vi "Acq-module5761.vi"(4 "NumChannels":u16, 5 "DMA number":i32, 6 "Selected Channels":T1[](array[typedef])=[enum."Empty", enum."Empty", enum."Empty", enum."Empty"], 7 "IntermediateFIFO":refnum<k21>="FIFO0", 8 "DebugActivation":bool, 9 "GroupEnableN":bool, 10 "SamplingRateN(DecimationFactor)":u16, 11 "DMATtoHOSTBlockNWords":u16) -> ()   [LabVIEW 2013, in "IRIO.lvlib"]
uses:
  IRIO.lvlib
  ctl/SelectedChannels.ctl
  <vilib>/rvi/DataTransferAndStorage/Container/Common/niFpgaContainerGetUniqueNameForEmu.vi
  <vilib>/rvi/DataTransferAndStorage/Container/Common/niFpgaContainerSetEmuInfo.vi
  <vilib>/rvi/eio/common/nirviEmuReportErrorAndStop.vi
  <vilib>/rvi/DataTransferAndStorage/Container/Common/niFpgaContainerExecOnDevCompGetState.vi
  <vilib>/rvi/DataTransferAndStorage/Register/Emulation/niFpgaRegisterEmulationFpgaImpl.vi
  <instcachedir>/1/niFpgaRegisterEmulationFpgaImpl_DCF4BC0110594B98B44A971D60CEEC4D.lvgen/niFpgaRegisterEmulationFpgaImpl_DCF4BC0110594B98B44A971D60CEEC4D_003.vi
  <instcachedir>/1/niFpgaRegisterEmulationFpgaImpl_DCF4BC0110594B98B44A971D60CEEC4D.lvgen/niFpgaRegisterEmulationFpgaImpl_DCF4BC0110594B98B44A971D60CEEC4D_005.vi
  <vilib>/rvi/eio/common/nirviEmuTemplateMethod_errors.vi
  common/GlobalReg.vi
  <instcachedir>/1/niFpgaRegisterEmulationFpgaImpl_DCF4BC0110594B98B44A971D60CEEC4D.lvgen/niFpgaRegisterEmulationFpgaImpl_DCF4BC0110594B98B44A971D60CEEC4D_004.vi
  <vilib>/rvi/FIFO/Fifo_Resource/nirvififoEmulationWriteFpgaImpl.vi
  <vilib>/rvi/interface/RandomDataEmulation/nirviRandomDataFPGAFIFO.vi
  <vilib>/rvi/interface/RandomDataEmulation/niFpgaRandomDataHandleErrors.vi
  <vilib>/rvi/Emulation/niFpgaSctlEmulationGetInTimedLoop.vi
  <vilib>/rvi/Emulation/niFpgaProcessEmulError.vi
  <vilib>/rvi/LocalResourceManager/LocalResourceManager.xnode
  <vilib>/rvi/DataTransferAndStorage/Container/XNode/niFpgaContainer.xnode
  <vilib>/rvi/DataTransferAndStorage/Register/Emulation/niFpgaRegisterEmulationRefIn.vi
  <vilib>/eio/EIONode/EIONode.xnode
  <vilib>/rvi/FIFO/Fifo_Resource/niFpgaFifoEmulationRefIn.vi
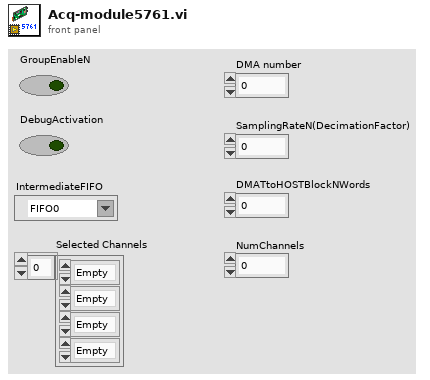
[diagram p1: front panel]
types:
  T1 = typedef "IRIO.lvlib/SelectedChannels.ctl" = enum16{"Empty", "AI0", "AI1", "AI2", "AI3", "SignalGenerator0", "SignalGenerator1", "DDCA_PORT0", "DDCA_PORT1", "DDCA_PORT2", "DDCB_PORT0", "DDCB_PORT1", "DDCB_PORT2"}
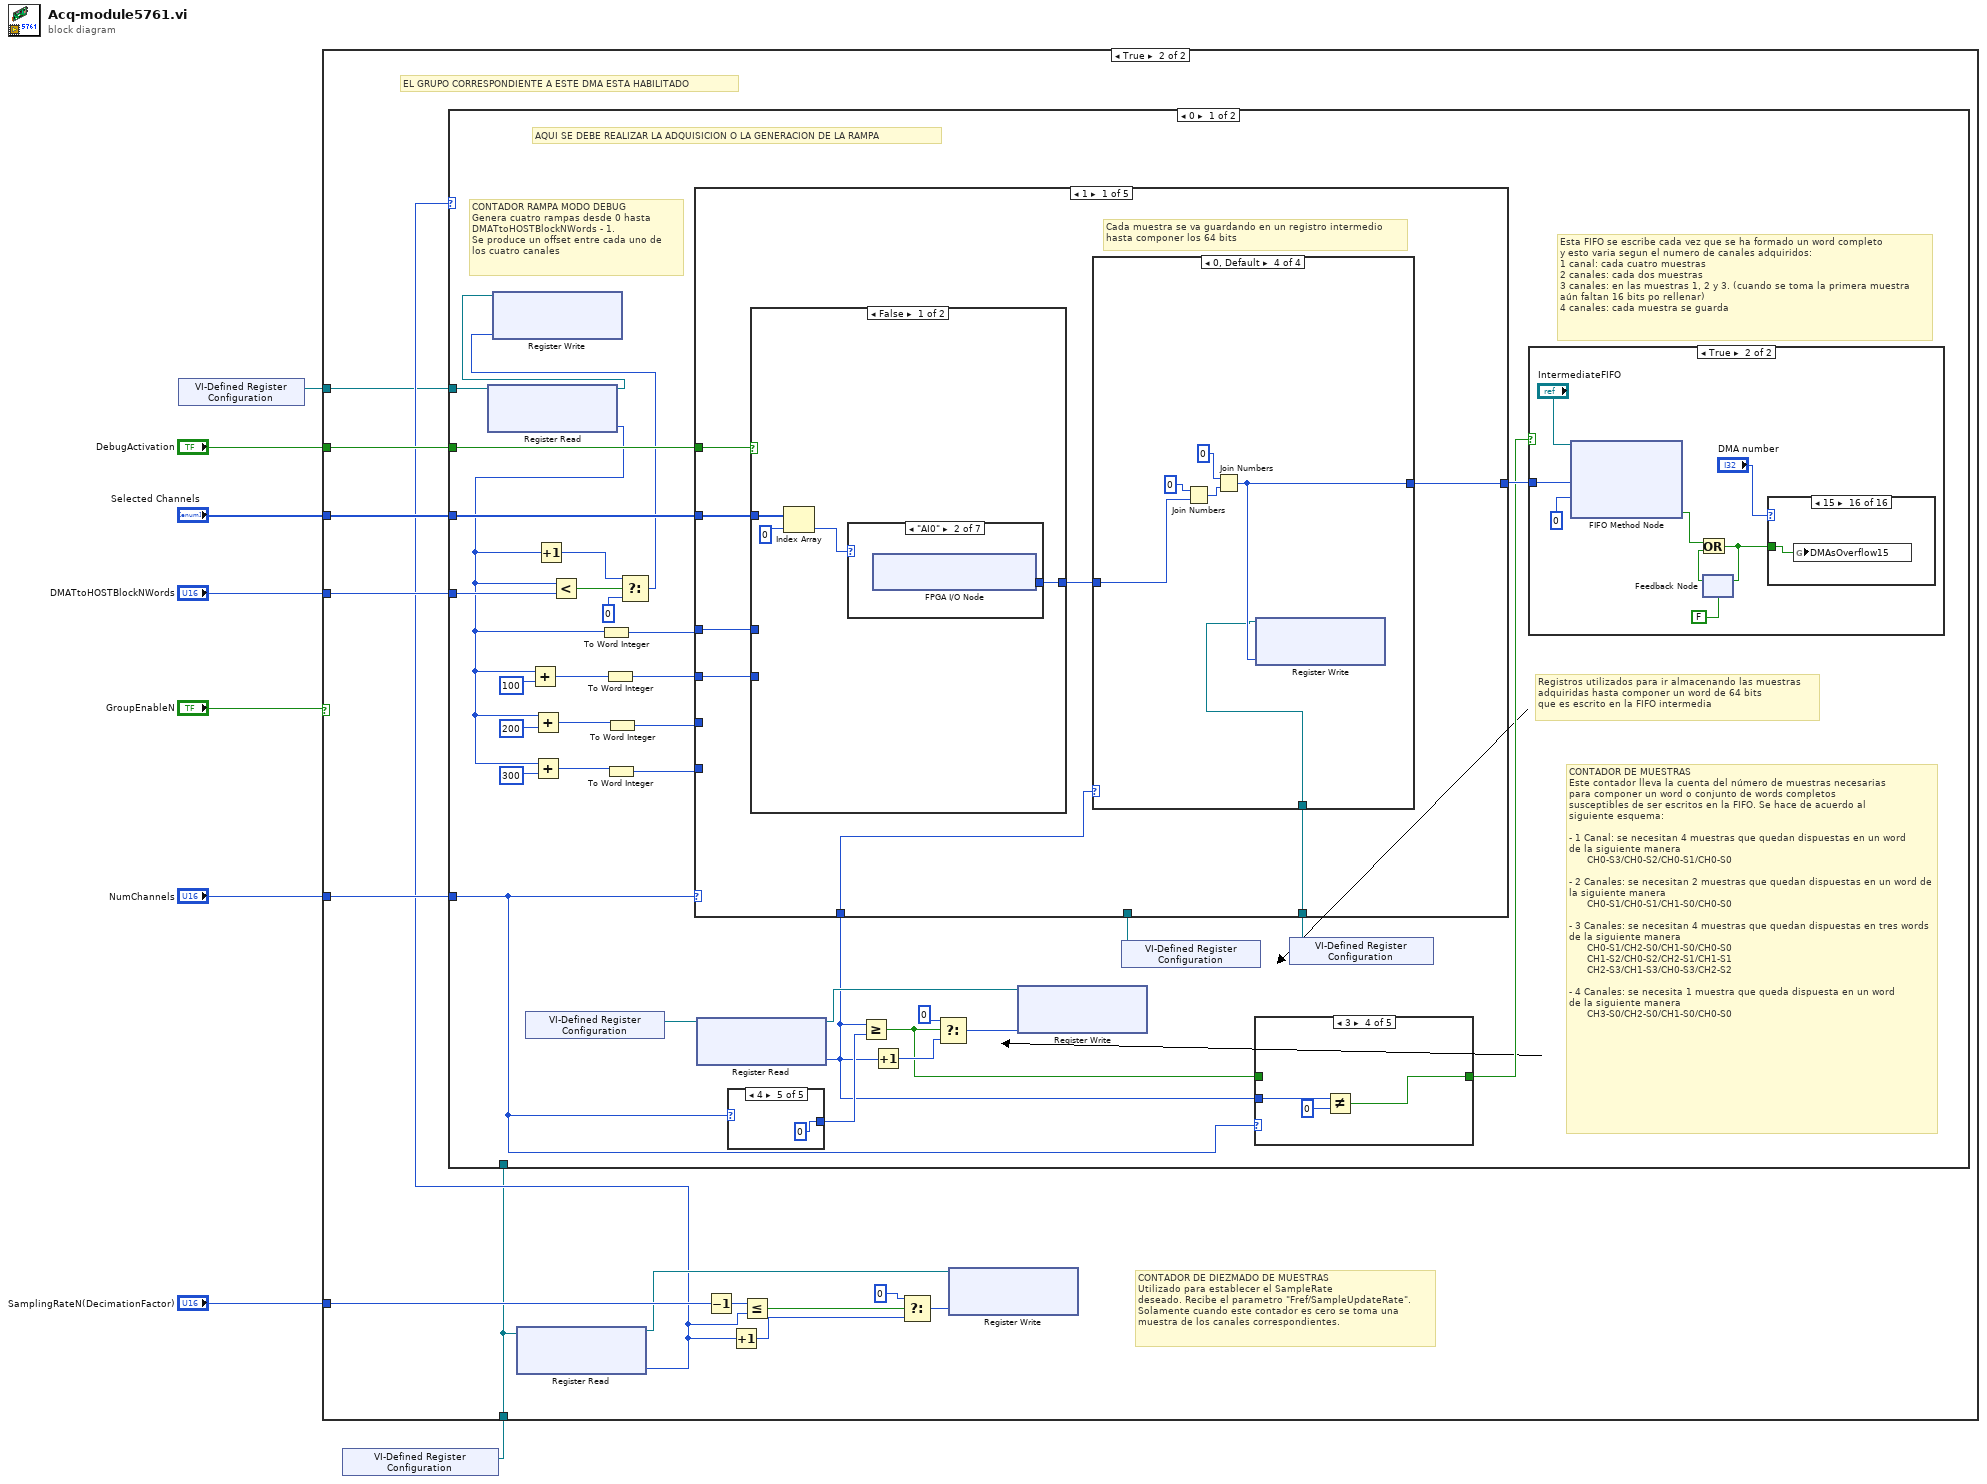
[diagram p0: block diagram]
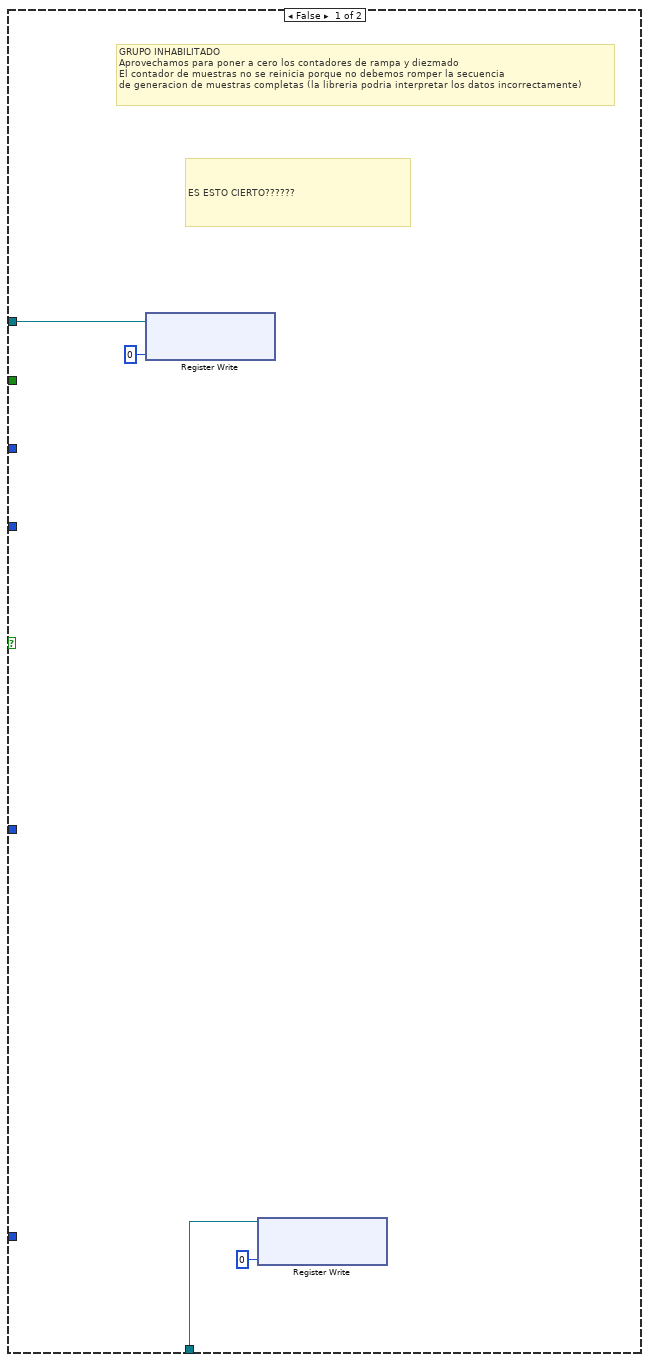
[diagram p2: hidden frame]
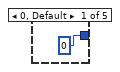
[diagram p7: hidden frame]
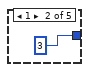
[diagram p8: hidden frame]
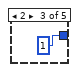
[diagram p9: hidden frame]
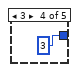
[diagram p10: hidden frame]
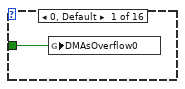
[diagram p12: hidden frame]
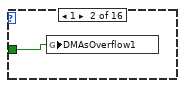
[diagram p13: hidden frame]
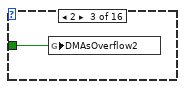
[diagram p14: hidden frame]
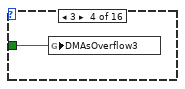
[diagram p15: hidden frame]
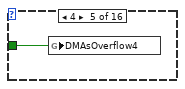
[diagram p16: hidden frame]
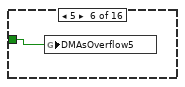
[diagram p17: hidden frame]
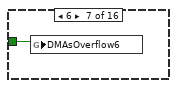
[diagram p18: hidden frame]
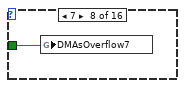
[diagram p19: hidden frame]
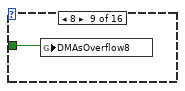
[diagram p20: hidden frame]
diagram:
  n1 = xnode ("VI-Defined Register Configuration")() -> ("Register Out"=w2:refnum<k21>)
  n2 = xnode ("VI-Defined Register Configuration")() -> ("Register Out"=w3:refnum<k21>)
  n3 = case shown="True" "GroupEnableN" {
    tunnel: "DebugActivation" -> [_ w26]
    tunnel: "DMATtoHOSTBlockNWords" -> [_ w25]
    tunnel: "NumChannels" -> [_ w24]
    tunnel: "Selected Channels" -> [_ w23]
    tunnel: "SamplingRateN(DecimationFactor)" -> [_ w18]
    tunnel: w3 -> [w12 w14]
    tunnel: w2 -> [w10 w13]
    frame False {
      # "ES ESTO CIERTO??????"
      # "GRUPO INHABILITADO\nAprovechamos para poner a cero los contadores de rampa y diezmado\nEl contador de muestras no se reinicia porque no debemos romper la secuencia\nde generacion de muestras completas (la libreria podria interpretar los datos incorrectamente)"
      n4 = xnode ("Register Write")("Data"=u16 0, "Register In"=w10) -> ()  [unwired: 1 out]
      n5 = xnode ("Register Write")("Data"=u16 0, "Register In"=w12) -> ()  [unwired: 1 out]
    }
    frame True {
      # "EL GRUPO CORRESPONDIENTE A ESTE DMA ESTA HABILITADO"
      # "CONTADOR DE DIEZMADO DE MUESTRAS\nUtilizado para establecer el SampleRate \ndeseado. Recibe el parametro \"Fref/SampleUpdateRate\".\nSolamente cuando este contador es cero se toma una\nmuestra de los canales correspondientes."
      n6 = xnode ("Register Read")("Register In"=w14) -> ("Register Out"=w17:refnum<k21>, "Data"=w15:u16)
      n7 = case shown="0" w15 {
        tunnel: w26 -> [w59 _]
        tunnel: w25 -> [w54 _]
        tunnel: w24 -> [w46 _]
        tunnel: w23 -> [w57 _]
        tunnel: w14 -> [_ _]
        tunnel: w13 -> [w39 _]
        frame 0 {
          # "Esta FIFO se escribe cada vez que se ha formado un word completo\ny esto varia segun el numero de canales adquiridos: \n1 canal: cada cuatro muestras\n2 canales: cada dos muestras\n3 canales: en las muestras 1, 2 y 3. (cuando se toma la primera muestra\naún faltan 16 bits po rellenar)\n4 canales: cada muestra se guarda"
          # "CONTADOR DE MUESTRAS\nEste contador lleva la cuenta del número de muestras necesarias\npara componer un word o conjunto de words completos\nsusceptibles de ser escritos en la FIFO. Se hace de acuerdo al\nsiguiente esquema:\n\n- 1 Canal: se necesitan 4 muestras que quedan dispuestas en un word \nde la siguiente manera\n      CH0-S3/CH0-S2/CH0-S1/CH0-S0\n\n- 2 Canales: se necesitan 2 muestras que quedan dispuestas en un word de la siguiente manera\n      CH0-S1/CH0-S1/CH1-S0/CH0-S0\n\n- 3 Canales: se necesitan 4 muestras que quedan dispuestas en tres words de la siguiente manera\n      CH0-S1/CH2-S0/CH1-S0/CH0-S0\n      CH1-S2/CH0-S2/CH2-S1/CH1-S1\n      CH2-S3/CH1-S3/CH0-S3/CH2-S2\n\n- 4 Canales: se necesita 1 muestra que queda dispuesta en un word \nde la siguiente manera\n      CH3-S0/CH2-S0/CH1-S0/CH0-S0"
          # "Registros utilizados para ir almacenando las muestras\nadquiridas hasta componer un word de 64 bits\nque es escrito en la FIFO intermedia"
          # "CONTADOR RAMPA MODO DEBUG\nGenera cuatro rampas desde 0 hasta \nDMATtoHOSTBlockNWords - 1.\nSe produce un offset entre cada uno de \nlos cuatro canales"
          # "AQUI SE DEBE REALIZAR LA ADQUISICION O LA GENERACION DE LA RAMPA"
          n8 = xnode ("Register Read")("Register In"=w39) -> ("Data"=w27:u16, "Register Out"=w38:refnum<k21>)
          n9 = xnode ("VI-Defined Register Configuration")() -> ("Register Out"=w42:refnum<k21>)
          n10 = Add(x=w27, y=u16 100) -> (x+y=w34:u16)
          n11 = Add(x=w27, y=u16 200) -> (x+y=w32:u16)
          n12 = Add(x=w27, y=u16 300) -> (x+y=w30:u16)
          n13 = Increment(x=w27) -> (x+1=w56:u16)
          n14 = Less?(x=w27, y=w54) -> (x < y?=w55:bool)
          n15 = To Word Integer(number=w27) -> (16bit integer=w35:i16)
          n16 = To Word Integer(number=w34) -> (16bit integer=w33:i16)
          n17 = To Word Integer(number=w30) -> (16bit integer=w29:i16)
          n18 = To Word Integer(number=w32) -> (16bit integer=w31:i16)
          n19 = Select(t=w56, s=w55, f=u16 0) -> (s? t:f=w37:u16)
          n20 = xnode ("Register Write")("Data"=w37, "Register In"=w38) -> ()  [unwired: 1 out]
          n21 = xnode ("Register Read")("Register In"=w42) -> ("Register Out"=w47:refnum<k21>, "Data"=w43:u8)
          n22 = case shown="4" w46 {
            tunnel: [u8 0 u8 3 u8 1 u8 3 u8 0] -> w48
            frame 0, Default {
            }
            frame 1 {
            }
            frame 2 {
            }
            frame 3 {
            }
            frame 4 {
            }
          }
          n23 = Greater Or Equal?(x=w43, y=w48) -> (x >= y?=w45:bool)
          n24 = Increment(x=w43) -> (x+1=w51:u8)
          n25 = Select(t=u8 0 ("f"), s=w45, f=w51) -> (s? t:f=w49:u8)
          n26 = xnode ("Register Write")("Data"=w49, "Register In"=w47) -> ()  [unwired: 1 out]
          n27 = xnode ("VI-Defined Register Configuration")() -> ("Register Out"=w41:refnum<k21>)
          n28 = case shown="3" w46 {
            tunnel: w45 -> [w60 w61 w62 _ w66]
            tunnel: [w60 w61 w62 w63 w66] -> w44
            tunnel: w43 -> [_ _ _ w65 _]
            frame 0, Default {
            }
            frame 1 {
            }
            frame 2 {
            }
            frame 3 {
              n29 = Not Equal?(x=w65, y=u8 0) -> (x != y?=w63:bool)
            }
            frame 4 {
            }
          }
          n30 = xnode ("VI-Defined Register Configuration")() -> ("Register Out"=w40:refnum<k21>)
          n31 = case shown="1" w46 {
            tunnel: w59 -> [w103 w155 w206 w305 _]
            tunnel: w35 -> [w100 w152 w203 w304 _]
            tunnel: [w101 w153 w204 w300 u64 0] -> w58
            tunnel: w57 -> [w102 w154 w205 w303 _]
            tunnel: w33 -> [w98 w149 w200 w296 _]
            tunnel: w31 -> [_ _ w198 w295 _]
            tunnel: w29 -> [_ _ _ w294 _]
            tunnel: w43 -> [w97 w148 w197 _ _]
            tunnel: w41 -> [_ _ w196 _ _]
            tunnel: w40 -> [w96 w147 w195 _ _]
            frame 1 {
              # "Cada muestra se va guardando en un registro intermedio\nhasta componer los 64 bits"
              n32 = case shown="False" w103 {
                tunnel: w102 -> [w105 _]
                tunnel: [w104 w117] -> w99
                tunnel: w100 -> [_ w117]
                tunnel: w98 -> [_ _]
                frame False {
                  n33 = Index Array(array=w105, index=0) -> (element=w106:T1)
                  n34 = case shown="\"AI0\"" w106 {
                    tunnel: [i16 0 ("IO Module\\AI 0") w109 w110 w111 w112 w114 w116] -> w104
                    frame "Empty", Default {
                    }
                    frame "AI0" {
                      n35 = xnode "FPGA I/O Node"() -> ("IO Module\\AI 0 Data N"=w109:i16)  [unwired: 1 in, 1 out]
                    }
                    frame "AI1" {
                      n36 = xnode "FPGA I/O Node"() -> ("IO Module\\AI 1 Data N"=w110:i16)  [unwired: 1 in, 1 out]
                    }
                    frame "AI2" {
                      n37 = xnode "FPGA I/O Node"() -> ("IO Module\\AI 2 Data N"=w111:i16)  [unwired: 1 in, 1 out]
                    }
                    frame "AI3" {
                      n38 = xnode "FPGA I/O Node"() -> ("IO Module\\AI 3 Data N"=w112:i16)  [unwired: 1 in, 1 out]
                    }
                    frame "SignalGenerator0" {
                      n39 = global read "GlobalReg.vi" "SimulatedAO0"() -> (w113:i32)
                      n40 = To Word Integer(number=w113) -> (16bit integer=w114:i16)
                    }
                    frame "SignalGenerator1" {
                      n41 = global read "GlobalReg.vi" "SimulatedAO1"() -> (w115:i32)
                      n42 = To Word Integer(number=w115) -> (16bit integer=w116:i16)
                    }
                  }
                }
                frame True {
                }
              }
              n43 = case shown="0, Default" w97 {
                tunnel: w99 -> [w120 w129 w136 w146]
                tunnel: [w119 w127 w134 w143] -> w101
                tunnel: w96 -> [w118 w126 w133 w141]
                frame 1 {
                  n44 = xnode ("Register Read")("Register In"=w118) -> ("Data"=w125:u64)  [unwired: 1 out]
                  n45 = Split Number(x=w125) -> (lo(x)=w124:u32)  [unwired: 1 out]
                  n46 = Split Number(x=w124) -> (lo(x)=w121:u16)  [unwired: 1 out]
                  n47 = Join Numbers(hi=w120, lo=w121) -> ((hi.lo)=w123:u32)
                  n48 = Join Numbers(hi=u32 0, lo=w123) -> ((hi.lo)=w119:u64)
                  n49 = xnode ("Register Write")("Data"=w119, "Register In"=w118) -> ()  [unwired: 1 out]
                }
                frame 2 {
                  n50 = xnode ("Register Read")("Register In"=w126) -> ("Data"=w132:u64)  [unwired: 1 out]
                  n51 = Split Number(x=w132) -> (lo(x)=w131:u32)  [unwired: 1 out]
                  n52 = Join Numbers(hi=u32 0, lo=w129) -> ((hi.lo)=w130:u64)
                  n53 = Join Numbers(hi=w130, lo=w131) -> ((hi.lo)=w127:u64)
                  n54 = xnode ("Register Write")("Data"=w127, "Register In"=w126) -> ()  [unwired: 1 out]
                }
                frame 3 {
                  n55 = xnode ("Register Read")("Register In"=w133) -> ("Data"=w140:u64)  [unwired: 1 out]
                  n56 = Split Number(x=w140) -> (hi(x)=w137:u32, lo(x)=w139:u32)
                  n57 = Split Number(x=w137) -> (lo(x)=w135:u16)  [unwired: 1 out]
                  n58 = Join Numbers(hi=w136, lo=w135) -> ((hi.lo)=w138:u32)
                  n59 = Join Numbers(hi=w138, lo=w139) -> ((hi.lo)=w134:u64)
                }
                frame 0, Default {
                  n60 = Join Numbers(hi=u16 0, lo=w146) -> ((hi.lo)=w145:u32)
                  n61 = Join Numbers(hi=u32 0, lo=w145) -> ((hi.lo)=w143:u64)
                  n62 = xnode ("Register Write")("Data"=w143, "Register In"=w141) -> ()  [unwired: 1 out]
                }
              }
            }
            frame 2 {
              # "Cada muestra de dos canales se van guardando en un registro\nintermedio hasta componer los 64 bits"
              n63 = case shown="False" w155 {
                tunnel: w154 -> [w160 _]
                tunnel: [w157 w181] -> w151
                tunnel: [w156 w180] -> w150
                tunnel: w152 -> [_ w181]
                tunnel: w149 -> [_ w180]
                frame False {
                  n64 = Index Array(array=w160, index #1=0 ("index")) -> (element #1=w159:T1, element #2=w158:T1)  [unwired: 1 in]
                  n65 = case shown="\"AI0\"" w159 {
                    tunnel: [i16 0 ("IO Module\\AI 0") w172 w173 w174 w175 w177 w179] -> w157
                    frame "Empty", Default {
                    }
                    frame "AI0" {
                      n66 = xnode "FPGA I/O Node"() -> ("IO Module\\AI 0 Data N"=w172:i16)  [unwired: 1 in, 1 out]
                    }
                    frame "AI1" {
                      n67 = xnode "FPGA I/O Node"() -> ("IO Module\\AI 1 Data N"=w173:i16)  [unwired: 1 in, 1 out]
                    }
                    frame "AI2" {
                      n68 = xnode "FPGA I/O Node"() -> ("IO Module\\AI 2 Data N"=w174:i16)  [unwired: 1 in, 1 out]
                    }
                    frame "AI3" {
                      n69 = xnode "FPGA I/O Node"() -> ("IO Module\\AI 3 Data N"=w175:i16)  [unwired: 1 in, 1 out]
                    }
                    frame "SignalGenerator0" {
                      n70 = global read "GlobalReg.vi" "SimulatedAO0"() -> (w176:i32)
                      n71 = To Word Integer(number=w176) -> (16bit integer=w177:i16)
                    }
                    frame "SignalGenerator1" {
                      n72 = global read "GlobalReg.vi" "SimulatedAO1"() -> (w178:i32)
                      n73 = To Word Integer(number=w178) -> (16bit integer=w179:i16)
                    }
                  }
                  n74 = case shown="\"AI0\"" w158 {
                    tunnel: [i16 0 ("IO Module\\AI 0") w163 w164 w165 w166 w168 w170] -> w156
                    frame "Empty", Default {
                    }
                    frame "AI0" {
                      n75 = xnode "FPGA I/O Node"() -> ("IO Module\\AI 0 Data N"=w163:i16)  [unwired: 1 in, 1 out]
                    }
                    frame "AI1" {
                      n76 = xnode "FPGA I/O Node"() -> ("IO Module\\AI 1 Data N"=w164:i16)  [unwired: 1 in, 1 out]
                    }
                    frame "AI2" {
                      n77 = xnode "FPGA I/O Node"() -> ("IO Module\\AI 2 Data N"=w165:i16)  [unwired: 1 in, 1 out]
                    }
                    frame "AI3" {
                      n78 = xnode "FPGA I/O Node"() -> ("IO Module\\AI 3 Data N"=w166:i16)  [unwired: 1 in, 1 out]
                    }
                    frame "SignalGenerator0" {
                      n79 = global read "GlobalReg.vi" "SimulatedAO0"() -> (w167:i32)
                      n80 = To Word Integer(number=w167) -> (16bit integer=w168:i16)
                    }
                    frame "SignalGenerator1" {
                      n81 = global read "GlobalReg.vi" "SimulatedAO1"() -> (w169:i32)
                      n82 = To Word Integer(number=w169) -> (16bit integer=w170:i16)
                    }
                  }
                }
                frame True {
                }
              }
              n83 = case shown="0, Default" w148 {
                tunnel: w151 -> [w188 w194]
                tunnel: w150 -> [w187 w193]
                tunnel: [w185 w190] -> w153
                tunnel: w147 -> [w182 w189]
                frame 1 {
                  n84 = xnode ("Register Read")("Register In"=w182) -> ("Data"=w186:u64)  [unwired: 1 out]
                  n85 = Join Numbers(hi=w187, lo=w188) -> ((hi.lo)=w183:u32)
                  n86 = Split Number(x=w186) -> (lo(x)=w184:u32)  [unwired: 1 out]
                  n87 = Join Numbers(hi=w183, lo=w184) -> ((hi.lo)=w185:u64)
                }
                frame 0, Default {
                  n88 = Join Numbers(hi=w193, lo=w194) -> ((hi.lo)=w192:u32)
                  n89 = Join Numbers(hi=u32 0, lo=w192) -> ((hi.lo)=w190:u64)
                  n90 = xnode ("Register Write")("Data"=w190, "Register In"=w189) -> ()  [unwired: 1 out]
                }
              }
            }
            frame 3 {
              # "Se necesitan dos registros porque las muestras de los tres canales\nen ocasiones quedan distribuidas entre dos word consecutivas. Cada\nuno de los tres words que se van generando se van escribiendo\nen la FIFO en el ciclo en el que se termina de componer"
              n91 = case shown="False" w206 {
                tunnel: w205 -> [w213 _]
                tunnel: [w209 w244] -> w202
                tunnel: [w208 w243] -> w201
                tunnel: w203 -> [_ w244]
                tunnel: w200 -> [_ w243]
                tunnel: [w207 w242] -> w199
                tunnel: w198 -> [_ w242]
                frame False {
                  n92 = Index Array(array=w213, index #1=0 ("index")) -> (element #1=w212:T1, element #2=w211:T1, element #3=w210:T1)  [unwired: 2 in]
                  n93 = case shown="\"AI0\"" w212 {
                    tunnel: [i16 0 ("IO Module\\AI 0") w234 w235 w236 w237 w239 w241] -> w209
                    frame "Empty", Default {
                    }
                    frame "AI0" {
                      n94 = xnode "FPGA I/O Node"() -> ("IO Module\\AI 0 Data N"=w234:i16)  [unwired: 1 in, 1 out]
                    }
                    frame "AI1" {
                      n95 = xnode "FPGA I/O Node"() -> ("IO Module\\AI 1 Data N"=w235:i16)  [unwired: 1 in, 1 out]
                    }
                    frame "AI2" {
                      n96 = xnode "FPGA I/O Node"() -> ("IO Module\\AI 2 Data N"=w236:i16)  [unwired: 1 in, 1 out]
                    }
                    frame "AI3" {
                      n97 = xnode "FPGA I/O Node"() -> ("IO Module\\AI 3 Data N"=w237:i16)  [unwired: 1 in, 1 out]
                    }
                    frame "SignalGenerator0" {
                      n98 = global read "GlobalReg.vi" "SimulatedAO0"() -> (w238:i32)
                      n99 = To Word Integer(number=w238) -> (16bit integer=w239:i16)
                    }
                    frame "SignalGenerator1" {
                      n100 = global read "GlobalReg.vi" "SimulatedAO1"() -> (w240:i32)
                      n101 = To Word Integer(number=w240) -> (16bit integer=w241:i16)
                    }
                  }
                  n102 = case shown="\"AI0\"" w211 {
                    tunnel: [i16 0 ("IO Module\\AI 0") w225 w226 w227 w228 w230 w232] -> w208
                    frame "Empty", Default {
                    }
                    frame "AI0" {
                      n103 = xnode "FPGA I/O Node"() -> ("IO Module\\AI 0 Data N"=w225:i16)  [unwired: 1 in, 1 out]
                    }
                    frame "AI1" {
                      n104 = xnode "FPGA I/O Node"() -> ("IO Module\\AI 1 Data N"=w226:i16)  [unwired: 1 in, 1 out]
                    }
                    frame "AI2" {
                      n105 = xnode "FPGA I/O Node"() -> ("IO Module\\AI 2 Data N"=w227:i16)  [unwired: 1 in, 1 out]
                    }
                    frame "AI3" {
                      n106 = xnode "FPGA I/O Node"() -> ("IO Module\\AI 3 Data N"=w228:i16)  [unwired: 1 in, 1 out]
                    }
                    frame "SignalGenerator0" {
                      n107 = global read "GlobalReg.vi" "SimulatedAO0"() -> (w229:i32)
                      n108 = To Word Integer(number=w229) -> (16bit integer=w230:i16)
                    }
                    frame "SignalGenerator1" {
                      n109 = global read "GlobalReg.vi" "SimulatedAO1"() -> (w231:i32)
                      n110 = To Word Integer(number=w231) -> (16bit integer=w232:i16)
                    }
                  }
                  n111 = case shown="\"AI0\"" w210 {
                    tunnel: [i16 0 ("IO Module\\AI 0") w216 w217 w218 w219 w221 w223] -> w207
                    frame "Empty", Default {
                    }
                    frame "AI0" {
                      n112 = xnode "FPGA I/O Node"() -> ("IO Module\\AI 0 Data N"=w216:i16)  [unwired: 1 in, 1 out]
                    }
                    frame "AI1" {
                      n113 = xnode "FPGA I/O Node"() -> ("IO Module\\AI 1 Data N"=w217:i16)  [unwired: 1 in, 1 out]
                    }
                    frame "AI2" {
                      n114 = xnode "FPGA I/O Node"() -> ("IO Module\\AI 2 Data N"=w218:i16)  [unwired: 1 in, 1 out]
                    }
                    frame "AI3" {
                      n115 = xnode "FPGA I/O Node"() -> ("IO Module\\AI 3 Data N"=w219:i16)  [unwired: 1 in, 1 out]
                    }
                    frame "SignalGenerator0" {
                      n116 = global read "GlobalReg.vi" "SimulatedAO0"() -> (w220:i32)
                      n117 = To Word Integer(number=w220) -> (16bit integer=w221:i16)
                    }
                    frame "SignalGenerator1" {
                      n118 = global read "GlobalReg.vi" "SimulatedAO1"() -> (w222:i32)
                      n119 = To Word Integer(number=w222) -> (16bit integer=w223:i16)
                    }
                  }
                }
                frame True {
                }
              }
              n120 = case shown="0, Default" w197 {
                tunnel: w202 -> [w254 w262 w274 w289]
                tunnel: w201 -> [w253 w257 w273 w284]
                tunnel: [w252 w268 w280 w292] -> w204
                tunnel: w199 -> [w249 w256 w272 w283]
                tunnel: w196 -> [w247 w261 w275 w288]
                tunnel: w195 -> [w245 w255 w269 w281]
                frame 0, Default {
                  # "No se lleva\nnada a la memoria\nde momento"
                  n121 = Join Numbers(hi=u32 0, lo=w249) -> ((hi.lo)=w250:u64)
                  n122 = Join Numbers(hi=w253, lo=w254) -> ((hi.lo)=w251:u32)
                  n123 = xnode ("Register Write")("Data"=u64 0, "Register In"=w247) -> ()  [unwired: 1 out]
                  n124 = Join Numbers(hi=w250, lo=w251) -> ((hi.lo)=w252:u64)
                  n125 = xnode ("Register Write")("Data"=w252, "Register In"=w245) -> ()  [unwired: 1 out]
                }
                frame 1 {
                  # "Listo registro 1"
                  n126 = Join Numbers(hi=w256, lo=w257) -> ((hi.lo)=w259:u32)
                  n127 = xnode ("Register Read")("Register In"=w255) -> ("Data"=w266:u64)  [unwired: 1 out]
                  n128 = Join Numbers(hi=u32 0, lo=w259) -> ((hi.lo)=w260:u64)
                  n129 = xnode ("Register Write")("Data"=w260, "Register In"=w261) -> ()  [unwired: 1 out]
                  n130 = Split Number(x=w266) -> (hi(x)=w264:u32, lo(x)=w265:u32)
                  n131 = Split Number(x=w264) -> (lo(x)=w263:u16)  [unwired: 1 out]
                  n132 = Join Numbers(hi=w262, lo=w263) -> ((hi.lo)=w267:u32)
                  n133 = Join Numbers(hi=w267, lo=w265) -> ((hi.lo)=w268:u64)
                }
                frame 2 {
                  w271 = u32 0 ("hi")
                  # "Listo registro 2"
                  n134 = Join Numbers(hi=w271, lo=w272) -> ((hi.lo)=w276:u64)
                  n135 = xnode ("Register Read")("Register In"=w275) -> ("Data"=w278:u64)  [unwired: 1 out]
                  n136 = Join Numbers(hi=w271, lo=w276) -> ((hi.lo)=w270:u64)
                  n137 = xnode ("Register Write")("Data"=w270, "Register In"=w269) -> ()  [unwired: 1 out]
                  n138 = Split Number(x=w278) -> (lo(x)=w277:u32)  [unwired: 1 out]
                  n139 = Join Numbers(hi=w273, lo=w274) -> ((hi.lo)=w279:u32)
                  n140 = Join Numbers(hi=w279, lo=w277) -> ((hi.lo)=w280:u64)
                }
                frame 3 {
                  # "Listo registro 1"
                  n141 = xnode ("Register Read")("Register In"=w281) -> ("Data"=w291:u64)  [unwired: 1 out]
                  n142 = xnode ("Register Write")("Data"=u32 0 ("hi"), "Register In"=w288) -> ()  [unwired: 1 out]
                  n143 = Split Number(x=w291) -> (lo(x)=w286:u32)  [unwired: 1 out]
                  n144 = Split Number(x=w286) -> (lo(x)=w290:u16)  [unwired: 1 out]
                  n145 = Join Numbers(hi=w283, lo=w284) -> ((hi.lo)=w282:u32)
                  n146 = Join Numbers(hi=w289, lo=w290) -> ((hi.lo)=w285:u32)
                  n147 = Join Numbers(hi=w282, lo=w285) -> ((hi.lo)=w292:u64)
                }
              }
            }
            frame 4 {
              # "Se compone un word completo con una\nsola muestra"
              n148 = case shown="False" w305 {
                tunnel: w304 -> [w309 _]
                tunnel: w303 -> [_ w318]
                tunnel: [w306 w313] -> w299
                tunnel: [w307 w312] -> w298
                tunnel: [w308 w311] -> w297
                tunnel: [w309 w310] -> w293
                tunnel: w296 -> [w308 _]
                tunnel: w295 -> [w307 _]
                tunnel: w294 -> [w306 _]
                frame True {
                }
                frame False {
                  # "CH0"
                  # "CH1"
                  # "CH2"
                  # "CH3"
                  n149 = Index Array(array=w318, index #1=0 ("index")) -> (element #1=w314:T1, element #2=w315:T1, element #3=w316:T1, element #4=w317:T1)  [unwired: 3 in]
                  n150 = case shown="\"AI0\"" w317 {
                    tunnel: [i16 0 ("IO Module\\AI 0") w348 w349 w350 w351 w353 w355] -> w313
                    frame "Empty", Default {
                    }
                    frame "AI0" {
                      n151 = xnode "FPGA I/O Node"() -> ("IO Module\\AI 0 Data N"=w348:i16)  [unwired: 1 in, 1 out]
                    }
                    frame "AI1" {
                      n152 = xnode "FPGA I/O Node"() -> ("IO Module\\AI 1 Data N"=w349:i16)  [unwired: 1 in, 1 out]
                    }
                    frame "AI2" {
                      n153 = xnode "FPGA I/O Node"() -> ("IO Module\\AI 2 Data N"=w350:i16)  [unwired: 1 in, 1 out]
                    }
                    frame "AI3" {
                      n154 = xnode "FPGA I/O Node"() -> ("IO Module\\AI 3 Data N"=w351:i16)  [unwired: 1 in, 1 out]
                    }
                    frame "SignalGenerator0" {
                      n155 = global read "GlobalReg.vi" "SimulatedAO0"() -> (w352:i32)
                      n156 = To Word Integer(number=w352) -> (16bit integer=w353:i16)
                    }
                    frame "SignalGenerator1" {
                      n157 = global read "GlobalReg.vi" "SimulatedAO1"() -> (w354:i32)
                      n158 = To Word Integer(number=w354) -> (16bit integer=w355:i16)
                    }
                  }
                  n159 = case shown="\"AI0\"" w316 {
                    tunnel: [i16 0 ("IO Module\\AI 0") w339 w340 w341 w342 w344 w346] -> w312
                    frame "Empty", Default {
                    }
                    frame "AI0" {
                      n160 = xnode "FPGA I/O Node"() -> ("IO Module\\AI 0 Data N"=w339:i16)  [unwired: 1 in, 1 out]
                    }
                    frame "AI1" {
                      n161 = xnode "FPGA I/O Node"() -> ("IO Module\\AI 1 Data N"=w340:i16)  [unwired: 1 in, 1 out]
                    }
                    frame "AI2" {
                      n162 = xnode "FPGA I/O Node"() -> ("IO Module\\AI 2 Data N"=w341:i16)  [unwired: 1 in, 1 out]
                    }
                    frame "AI3" {
                      n163 = xnode "FPGA I/O Node"() -> ("IO Module\\AI 3 Data N"=w342:i16)  [unwired: 1 in, 1 out]
                    }
                    frame "SignalGenerator0" {
                      n164 = global read "GlobalReg.vi" "SimulatedAO0"() -> (w343:i32)
                      n165 = To Word Integer(number=w343) -> (16bit integer=w344:i16)
                    }
                    frame "SignalGenerator1" {
                      n166 = global read "GlobalReg.vi" "SimulatedAO1"() -> (w345:i32)
                      n167 = To Word Integer(number=w345) -> (16bit integer=w346:i16)
                    }
                  }
                  n168 = case shown="\"AI0\"" w315 {
                    tunnel: [i16 0 ("IO Module\\AI 0") w330 w331 w332 w333 w335 w337] -> w311
                    frame "Empty", Default {
                    }
                    frame "AI0" {
                      n169 = xnode "FPGA I/O Node"() -> ("IO Module\\AI 0 Data N"=w330:i16)  [unwired: 1 in, 1 out]
                    }
                    frame "AI1" {
                      n170 = xnode "FPGA I/O Node"() -> ("IO Module\\AI 1 Data N"=w331:i16)  [unwired: 1 in, 1 out]
                    }
                    frame "AI2" {
                      n171 = xnode "FPGA I/O Node"() -> ("IO Module\\AI 2 Data N"=w332:i16)  [unwired: 1 in, 1 out]
                    }
                    frame "AI3" {
                      n172 = xnode "FPGA I/O Node"() -> ("IO Module\\AI 3 Data N"=w333:i16)  [unwired: 1 in, 1 out]
                    }
                    frame "SignalGenerator0" {
                      n173 = global read "GlobalReg.vi" "SimulatedAO0"() -> (w334:i32)
                      n174 = To Word Integer(number=w334) -> (16bit integer=w335:i16)
                    }
                    frame "SignalGenerator1" {
                      n175 = global read "GlobalReg.vi" "SimulatedAO1"() -> (w336:i32)
                      n176 = To Word Integer(number=w336) -> (16bit integer=w337:i16)
                    }
                  }
                  n177 = case shown="\"AI0\"" w314 {
                    tunnel: [i16 0 ("IO Module\\AI 0") w321 w322 w323 w324 w326 w328] -> w310
                    frame "Empty", Default {
                    }
                    frame "AI0" {
                      n178 = xnode "FPGA I/O Node"() -> ("IO Module\\AI 0 Data N"=w321:i16)  [unwired: 1 in, 1 out]
                    }
                    frame "AI1" {
                      n179 = xnode "FPGA I/O Node"() -> ("IO Module\\AI 1 Data N"=w322:i16)  [unwired: 1 in, 1 out]
                    }
                    frame "AI2" {
                      n180 = xnode "FPGA I/O Node"() -> ("IO Module\\AI 2 Data N"=w323:i16)  [unwired: 1 in, 1 out]
                    }
                    frame "AI3" {
                      n181 = xnode "FPGA I/O Node"() -> ("IO Module\\AI 3 Data N"=w324:i16)  [unwired: 1 in, 1 out]
                    }
                    frame "SignalGenerator0" {
                      n182 = global read "GlobalReg.vi" "SimulatedAO0"() -> (w325:i32)
                      n183 = To Word Integer(number=w325) -> (16bit integer=w326:i16)
                    }
                    frame "SignalGenerator1" {
                      n184 = global read "GlobalReg.vi" "SimulatedAO1"() -> (w327:i32)
                      n185 = To Word Integer(number=w327) -> (16bit integer=w328:i16)
                    }
                  }
                }
              }
              n186 = Join Numbers(hi=w299, lo=w298) -> ((hi.lo)=w302:u32)
              n187 = Join Numbers(hi=w297, lo=w293) -> ((hi.lo)=w301:u32)
              n188 = Join Numbers(hi=w302, lo=w301) -> ((hi.lo)=w300:u64)
            }
            frame Default {
            }
          }
          n189 = case shown="True" w44 {
            tunnel: w58 -> [_ w74]
            frame False {
            }
            frame True {
              n190 = xnode ("FIFO Method Node")("Element"=w74, "Timeout"=0, "FIFO In"="IntermediateFIFO") -> ("Timed Out?"=w75:bool)  [unwired: 1 out]
              n191 = feedback #1(FALSE) -> (w77:bool)
              n192 = Or(x=w75, y=w77) -> (x .or. y?=w76:bool)
              n193 = feedback-in #1(w76) -> ()
              n194 = case shown="15" "DMA number" {
                tunnel: w76 -> [w80 w81 w82 w83 w84 w85 w86 w87 w88 w89 w90 w91 w92 w93 w94 w95]
                frame 0, Default {
                  n195 = global write "GlobalReg.vi" "DMAsOverflow0"(w80) -> ()
                }
                frame 1 {
                  n196 = global write "GlobalReg.vi" "DMAsOverflow1"(w81) -> ()
                }
                frame 2 {
                  n197 = global write "GlobalReg.vi" "DMAsOverflow2"(w82) -> ()
                }
                frame 3 {
                  n198 = global write "GlobalReg.vi" "DMAsOverflow3"(w83) -> ()
                }
                frame 4 {
                  n199 = global write "GlobalReg.vi" "DMAsOverflow4"(w84) -> ()
                }
                frame 5 {
                  n200 = global write "GlobalReg.vi" "DMAsOverflow5"(w85) -> ()
                }
                frame 6 {
                  n201 = global write "GlobalReg.vi" "DMAsOverflow6"(w86) -> ()
                }
                frame 7 {
                  n202 = global write "GlobalReg.vi" "DMAsOverflow7"(w87) -> ()
                }
                frame 8 {
                  n203 = global write "GlobalReg.vi" "DMAsOverflow8"(w88) -> ()
                }
                frame 9 {
                  n204 = global write "GlobalReg.vi" "DMAsOverflow9"(w89) -> ()
                }
                frame 10 {
                  n205 = global write "GlobalReg.vi" "DMAsOverflow10"(w90) -> ()
                }
                frame 11 {
                  n206 = global write "GlobalReg.vi" "DMAsOverflow11"(w91) -> ()
                }
                frame 12 {
                  n207 = global write "GlobalReg.vi" "DMAsOverflow12"(w92) -> ()
                }
                frame 13 {
                  n208 = global write "GlobalReg.vi" "DMAsOverflow13"(w93) -> ()
                }
                frame 14 {
                  n209 = global write "GlobalReg.vi" "DMAsOverflow14"(w94) -> ()
                }
                frame 15 {
                  n210 = global write "GlobalReg.vi" "DMAsOverflow15"(w95) -> ()
                }
              }
            }
          }
        }
        frame 1, Default {
        }
      }
      n211 = Decrement(x=w18) -> (x-1=w19:u16)
      n212 = Increment(x=w15) -> (x+1=w21:u16)
      n213 = Less Or Equal?(x=w19, y=w15) -> (x <= y?=w22:bool)
      n214 = Select(t=u16 0, s=w22, f=w21) -> (s? t:f=w16:u16)
      n215 = xnode ("Register Write")("Data"=w16, "Register In"=w17) -> ()  [unwired: 1 out]
    }
  }
